vi "AutoFollowAbsoluteTrajectoryNEWCommandInterrupt.vi"(6 "commandstarttime":dbl, 7 "command":string, 8 "error in (no error)":errorcluster, 9 "TimeOut (s)":dbl, 10 "End Orientation":dbl, 11 "Trajectory":T1 {"States"."POSE"."ROTATION"."SIN" format="%13.4f"; "States"."POSE"."ROTATION"."COS" format="%13.4f"; "States"."POSE"."ROTATION"."VALUE" format="%13.4f"; "States"."POSE"."TRANSLATION"."Y" format="%14.3f"; "States"."POSE"."TRANSLATION"."X" format="%14.3f"; "TotalTImeSecs" format="%20.3f"}) -> (0 "error out":errorcluster)   [LabVIEW 2023]
doc: "Wrapper class for drive straight"
uses:
  <vilib>/Rock Robotics/WPI/ThirdParty/JAS_Junk/TrajLib/TypeDef/TRAJECTORY.ctl
  <vilib>/Rock Robotics/WPI/ThirdParty/JAS_Junk/TrajLib/TypeDef/TRAJ_STATE.ctl
  <vilib>/Rock Robotics/WPI/ThirdParty/JAS_Junk/TrajLib/TypeDef/POSE2D.ctl
  <vilib>/Rock Robotics/WPI/ThirdParty/JAS_Junk/TrajLib/TypeDef/TRANSLATION2D.ctl
  <vilib>/Rock Robotics/WPI/ThirdParty/JAS_Junk/TrajLib/TypeDef/ROTATION2D.ctl
  <vilib>/Rock Robotics/WPI/ThirdParty/JAS_Junk/TrajLib/ChassisSpeeds_New.vi
  <vilib>/Rock Robotics/WPI/ThirdParty/JAS_Junk/TrajLib/Conv_Feet_Meters.vi
  <vilib>/Rock Robotics/WPI/ThirdParty/JAS_Junk/TrajLib/Conv_Deg_Radians.vi
  <vilib>/Utility/semaphor.llb/Obtain Semaphore Reference.vi
  <vilib>/Rock Robotics/WPI/ThirdParty/JAS_Junk/TrajLib/Timer_Reset.vi
  Drive/DriveGlobal.vi
  <vilib>/Rock Robotics/WPI/ThirdParty/JAS_Junk/TrajLib/Trajectory_Library.lvlib
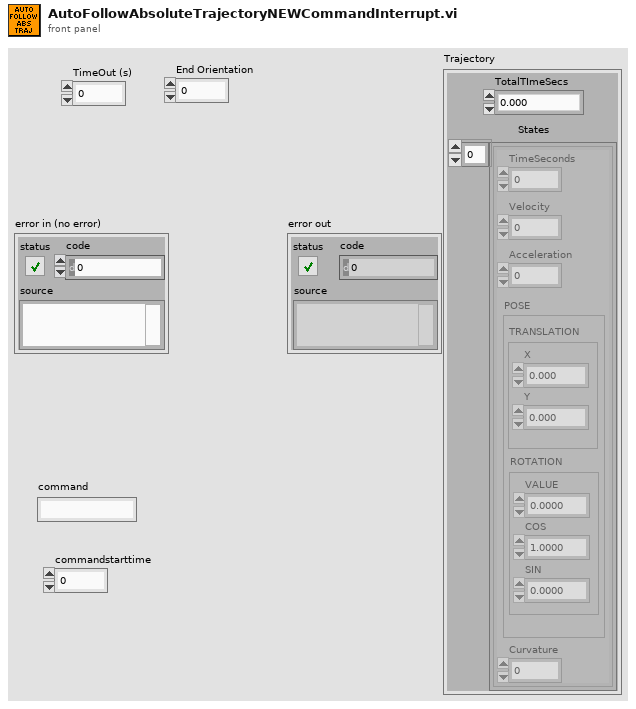
[diagram p1: front panel]
types:
  T1 = typedef "Trajectory_Library.lvlib/TRAJECTORY.ctl" = cluster{"TotalTImeSecs":dbl, "States":T2[]}
  T2 = typedef "Trajectory_Library.lvlib/TRAJ_STATE.ctl" = cluster{"TimeSeconds":dbl, "Velocity":dbl, "Acceleration":dbl, "POSE":T3, "Curvature":dbl}
  T3 = typedef "Trajectory_Library.lvlib/POSE2D.ctl" = cluster{"TRANSLATION":T4, "ROTATION":T5}
  T4 = typedef "Trajectory_Library.lvlib/TRANSLATION2D.ctl" = cluster{"X":dbl, "Y":dbl}
  T5 = typedef "Trajectory_Library.lvlib/ROTATION2D.ctl" = cluster{"VALUE":dbl, "COS":dbl, "SIN":dbl}
  T6 = typedef "Trajectory_Library.lvlib/TIMER.ctl" = cluster{"StartTime":dbl, "Accumulated TIme":dbl, "Running":bool, "semaphore":T7}
  T7 = typedef "Semaphore RefNum" = refnum<k1>
  T8 = typedef "Trajectory_Library.lvlib/CHASSIS_SPEEDS.ctl" = cluster{"vX":dbl, "vY":dbl, "vOmega":dbl}
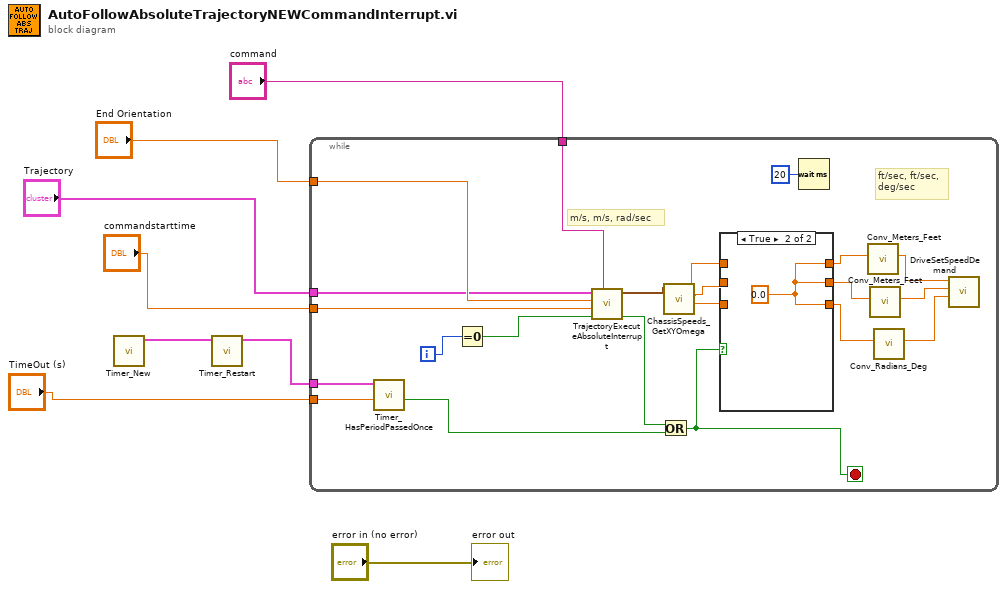
[diagram p0: block diagram]
diagram:
  n1 = call <vilib>:"Timer_New.vi"() -> ("TIMER"=w2:T6)  [unwired: 11 in]
  n2 = call <vilib>:"Timer_Restart.vi"("in Timer"=w2) -> ("out Timer"=w1:T6)  [unwired: 10 in]
  n3 = while {
    tunnel: w1 -> [w29]
    tunnel: "TimeOut (s)" -> [w28]
    tunnel: "Trajectory" -> [w11]
    tunnel: "End Orientation" -> [w12]
    tunnel: "commandstarttime" -> [w10]
    tunnel: "command" -> [w9]
    i -> [w30]
    stop <- w16 stop-if-true
    # "ft/sec, ft/sec,\ndeg/sec"
    # "m/s, m/s, rad/sec"
    n4 = call <vilib>:"Timer_HasPeriodPassedOnce.vi"("Period"=w28, "in Timer"=w29) -> ("Expired"=w27:bool)  [unwired: 7 in, 2 out]
    n5 = Equal To 0?(x=w30) -> (x = 0?=w13:bool)
    n6 = call "TrajectoryExecuteAbsoluteInterrupt.vi"("command"=w9, "Init"=w13, "commandstarttime"=w10, "End Abs\nOrientation Deg"=w12, "Trajectory"=w11) -> ("AtReference"=w15:bool, "Chassis Velocity Target"=w14:T8)  [unwired: 5 in]
    n7 = Or(x=w15, y=w27) -> (x .or. y?=w16:bool)
    n8 = call <vilib>:"ChassisSpeeds_GetXYOmega.vi"("CHASSIS"=w14) -> ("vAngular"=w25:dbl, "vY"=w24:dbl, "vX"=w23:dbl)  [unwired: 8 in]
    n9 = case shown="True" w16 {
      tunnel: w23 -> [w33 _]
      tunnel: w24 -> [w32 _]
      tunnel: w25 -> [w31 _]
      tunnel: [w33 w34] -> w22
      tunnel: [w32 w34] -> w20
      tunnel: [w31 w34] -> w18
      frame False {
      }
      frame True {
        w34 = 0.0 ("XSpeedDemand")
      }
    }
    n10 = Wait (ms)(milliseconds to wait=u32 20) -> ()  [unwired: 1 out]
    n11 = call <vilib>:"Conv_Meters_Feet.vi"("Meters"=w22) -> ("Feet"=w21:dbl)  [unwired: 10 in]
    n12 = call <vilib>:"Conv_Meters_Feet.vi"("Meters"=w20) -> ("Feet"=w19:dbl)  [unwired: 10 in]
    n13 = call <vilib>:"Conv_Radians_Deg.vi"("Radians"=w18) -> ("Degrees"=w17:dbl)  [unwired: 10 in]
    n14 = call "DriveSetSpeedDemand.vi"("ASpeedDemand (d/s)"=w17, "YSpeedDemand (ft/s)"=w19, "XSpeedDemand (ft/s)"=w21) -> ()  [unwired: 9 in]
  }
  "error out" <- "error in (no error)"
